vi "Com Write.vi"(8 "错误输入（无错误）":errorcluster, 10 "Wbuff":string, 11 "VISA In":refnum<visa-resource-name>) -> (0 "错误输出":errorcluster, 2 "START":string, 3 "VISA Out":refnum<visa-resource-name>)   [LabVIEW 2015, in "WZ5005E.lvlib"]
uses:
  <vilib>/Instr/_visa.llb/VISA Flush IO Buffer Mask.ctl
  WZ5005E.lvlib
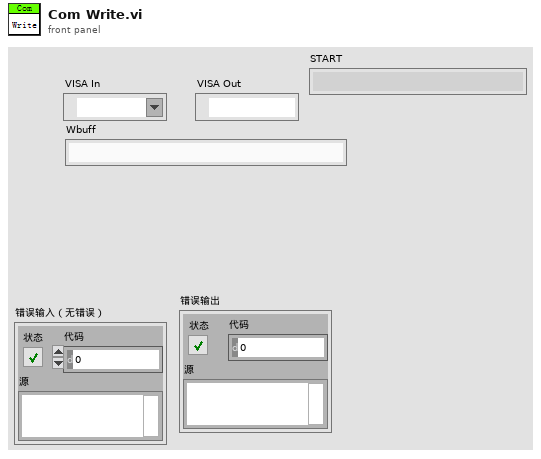
[diagram p1: front panel]
types:
  T1 = typedef "VISA Flush IO Buffer Mask.ctl" = u16
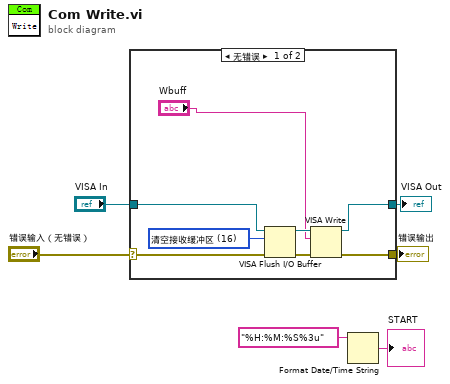
[diagram p0: block diagram]
diagram:
  n1 = case shown="无错误" "错误输入（无错误）" {
    selector: "错误输入（无错误）" -> [w9 w16]
    tunnel: "VISA In" -> [w14 w15]
    tunnel: [w10 w16] -> w5
    tunnel: [w8 w15] -> w3
    frame No Error {
      w12 = T1 16 items=["清空接收缓冲区"=16, "向设备写入传输缓冲区"=32, "清空接收缓冲区（无I/O）"=64, "清空传输缓冲区"=128] ("Mask")
      n2 = VISA Flush I/O Buffer(VISA resource name=w14, mask (16)=w12, error in (no error)=w9) -> (VISA resource name out=w13:refnum<visa-resource-name>, error out=w11:errorcluster)
      n3 = VISA Write(VISA resource name=w13, write buffer="Wbuff", error in (no error)=w11) -> (VISA resource name out=w8:refnum<visa-resource-name>, error out=w10:errorcluster)  [unwired: 1 out]
    }
    frame Error {
    }
  }
  "错误输出" <- w5
  "VISA Out" <- w3
  n4 = Format Date/Time String(time format string (%c)="%H:%M:%S%3u" ("时间格式字符串(%c)")) -> (date/time string=→"START":string)  [unwired: 2 in]
